vi "Retrieve AI DAQ Timestamp.vi"(8 "error in (no error)":errorcluster, 10 "AI TaskName":string, 11 "DaqData dCVT":T1) -> (0 "error out":errorcluster, 1 "found":bool, 2 "Timestamp":dbl, 3 "DaqData dCVT out":T1)   [LabVIEW 2017, in "DAQ.lvclass"]
doc: "Developed by Kevin Thompson\nkevin@thompsonengineering.net\n\nCopyright 2018-2020\nThompson Engineering, LLC\nAI scan timestamp is stored with IOName \"%sScanTS\" in DAQ Data Dict\n(%s = ['AI' | 'DI'])"
uses:
  DAQ.lvclass
  <vilib>/TELLC/Dynamic CVT API/TD Dynamic CVT DVR--ref.ctl
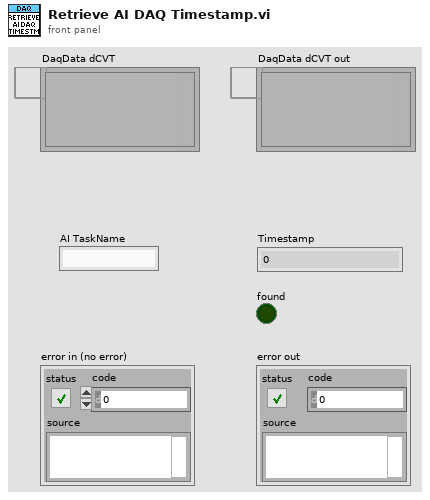
[diagram p1: front panel]
types:
  T1 = typedef "TD Dynamic CVT DVR--ref.ctl" = refnum<data-value>
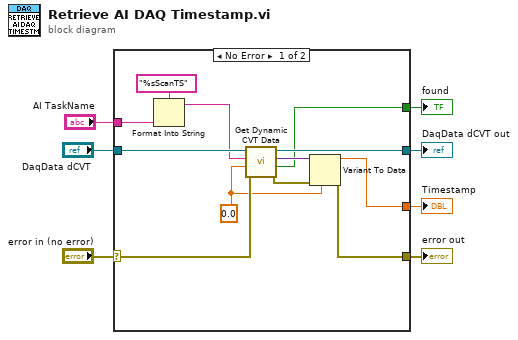
[diagram p0: block diagram]
diagram:
  n1 = case shown="No Error" "error in (no error)" {
    selector: "error in (no error)" -> [w17 w20]
    tunnel: [w9 w20] -> w7
    tunnel: [w19 w21] -> w6
    tunnel: "DaqData dCVT" -> [w18 w21]
    tunnel: [w11 _] -> w3
    tunnel: "AI TaskName" -> [w16 _]
    tunnel: [w8 _] -> w1
    frame No Error {
      w12 = 0.0 ("timestamp in")
      n2 = Format Into String(format string="%sScanTS" ("initial string"), w16) -> (resulting string=w14:string)  [unwired: 2 in, 1 out]
      n3 = call <vilib>:"Get Dynamic CVT Data.vi"("error in (no error)"=w17, "default value (empty variant)"=w12, "DataName"=w14, "dCVT DVR"=w18) -> ("error out"=w10:errorcluster, "found"=w8:bool, "value"=w13:variant, "dCVT DVR out"=w19:T1)  [unwired: 4 in]
      n4 = Variant To Data(error in=w10, type=w12, Variant=w13) -> (data=w11:dbl, error out=w9:errorcluster)
    }
    frame Error {
    }
  }
  "error out" <- w7
  "DaqData dCVT out" <- w6
  "Timestamp" <- w3
  "found" <- w1
